vi "GetAL.vi"(3 "error in (no error)":errorcluster, 5 "VISA resource":refnum<visa-resource-name>="COM1") -> (0 "error out":errorcluster, 1 "AL(=DSR) State":i16 min=0 max=1 step=1, 2 "dup VISA resource":refnum<visa-resource-name>="COM1")   [LabVIEW 2023]
doc: "Read state of the AL \nsignal from AVS-47B"
panel:
  # "GetAL.vi"
  # "This VI reads  the state (1 or 0)  of the AL  (Alarm)  Picobus input  line  (DSR  handshake of RS232). The Al signal is presently used only for indicating completion of an A/D conversion."
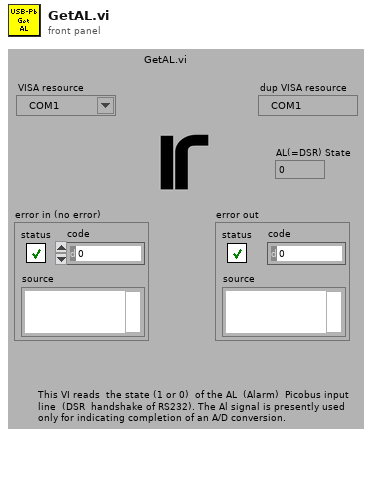
[diagram p1: front panel]
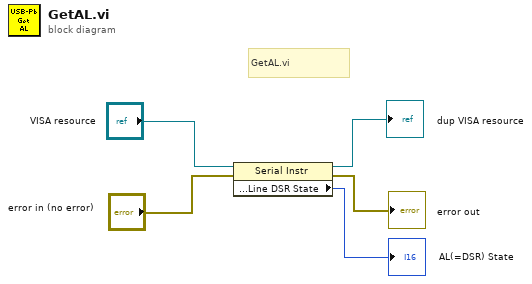
[diagram p0: block diagram]
diagram:
  # "GetAL.vi"
  n1 = property class="Serial Instr"(reference="VISA resource", error in="error in (no error)") -> (reference out=→"dup VISA resource":refnum<visa-resource-name>, error out=→"error out":errorcluster, "Serial Settings:Modem Line Settings:Line DSR State"=→"AL(=DSR) State":i16)
